vi "StartStop.vi"(8 "error in (no error)":errorcluster, 10 "Start/Stop":bool, 11 "Measurement Señal Actualizable in":refnum<class "Measurement Señal Actualizable.lvclass">) -> (0 "error out":errorcluster, 3 "Measurement Señal Actualizable out":refnum<class "Measurement Señal Actualizable.lvclass">)   [LabVIEW 2020, in "Measurement Señal Actualizable.lvlib" / "Measurement Señal Actualizable.lvclass"]
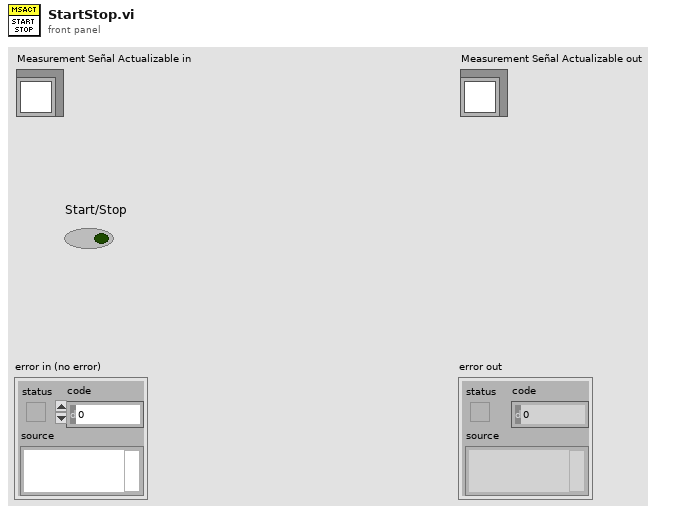
[diagram p1: front panel]
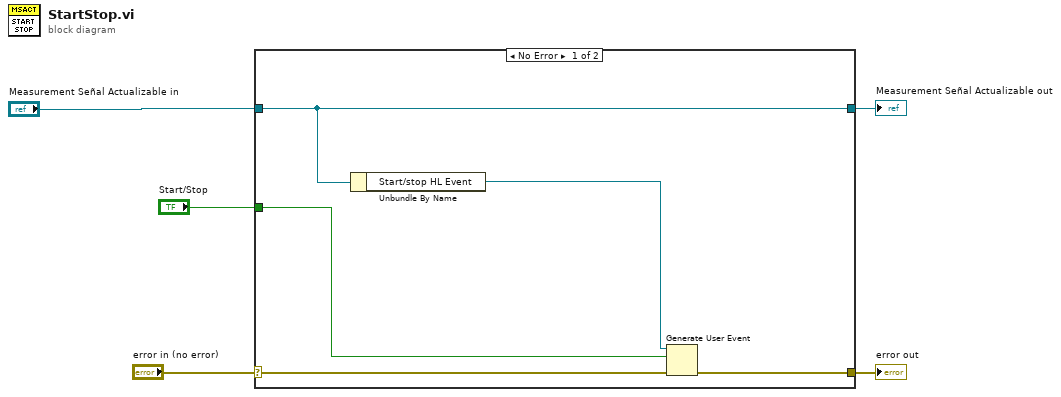
[diagram p0: block diagram]
diagram:
  n1 = case shown="No Error" "error in (no error)" {
    selector: "error in (no error)" -> [w10 w12]
    tunnel: [w8 w12] -> w4
    tunnel: [w9 w11] -> w2
    tunnel: "Measurement Señal Actualizable in" -> [w9 w11]
    tunnel: "Start/Stop" -> [w6 _]
    frame No Error {
      n2 = Unbundle By Name(w9) -> ("Start/stop HL Event"=w7:refnum<user-event>)
      n3 = Generate User Event(user event=w7, event data cluster=w6, error in=w10) -> (error out=w8:errorcluster)  [unwired: 1 in, 1 out]
    }
    frame Error {
    }
  }
  "error out" <- w4
  "Measurement Señal Actualizable out" <- w2
